vi "231106_Nikon_Led.vi"(8 "error in":errorcluster, 11 "Light path":u16(ring) items=["1- Eyepiece"=1, "2- Right"=2, "3- Left + Eyepiece"=3, "4- Left"=4]) -> (0 "error out":errorcluster, 3 "Cluster µscope":T1)   [LabVIEW 2014]
doc: "Ce VI permet d'afficher les LEDs en fonction du lightpath d'entrée.\nC'est purement visuel."
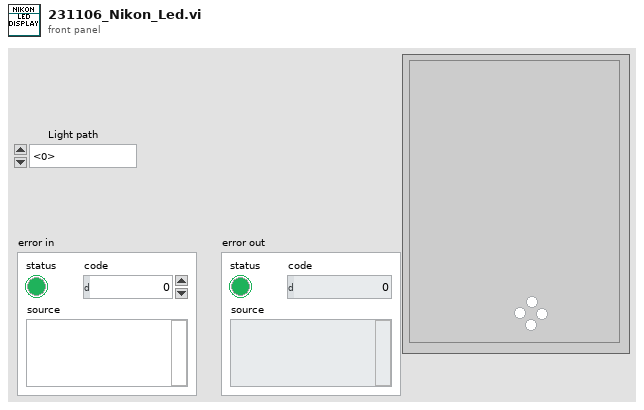
[diagram p1: front panel]
types:
  T1 = cluster{"Eyepiece":bool, "Right":bool, "Left + Eyepiece":bool, "Left":bool}
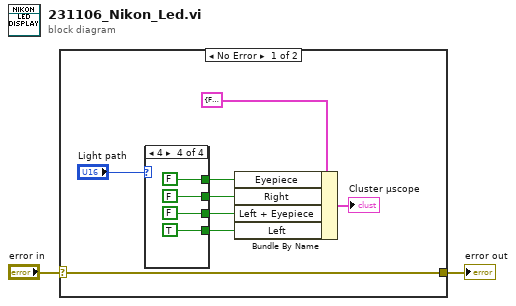
[diagram p0: block diagram]
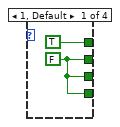
[diagram p2: hidden frame]
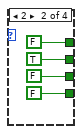
[diagram p3: hidden frame]
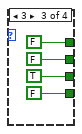
[diagram p4: hidden frame]
diagram:
  n1 = case shown="No Error" "error in" {
    selector: "error in" -> [w9 w25]
    tunnel: [w9 w25] -> w1
    frame No Error {
      n2 = case shown="4" "Light path" {
        tunnel: [TRUE FALSE FALSE FALSE] -> w7
        tunnel: [w11 TRUE FALSE FALSE] -> w6
        tunnel: [w11 FALSE TRUE FALSE] -> w5
        tunnel: [w11 FALSE FALSE TRUE] -> w4
        frame 1, Default {
          w11 = FALSE
        }
        frame 2 {
        }
        frame 3 {
        }
        frame 4 {
        }
      }
      n3 = Bundle By Name(cluster=T1 {"Eyepiece"=FALSE, "Right"=FALSE, "Left + Eyepiece"=FALSE, "Left"=FALSE} ("Cluster µscope 2"), "Eyepiece"=w7, "Right"=w6, "Left + Eyepiece"=w5, "Left"=w4) -> (→"Cluster µscope":T1)
    }
    frame Error {
    }
  }
  "error out" <- w1
